vi "X_plus_h.vi"(5 "X":dbl[](array[numeric]), 7 "h":dbl, 9 "i":i32) -> (6 "Xi+h":dbl[](array[numeric]))   [LabVIEW 2017, in "NI_Gmath.lvlib"]
uses:
  <vilib>/gmath/NI_Gmath.lvlib
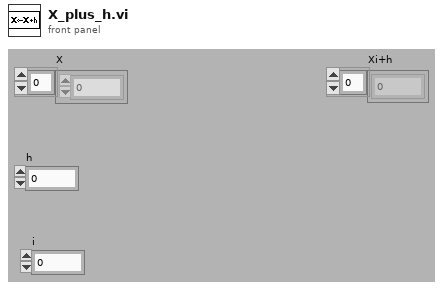
[diagram p1: front panel]
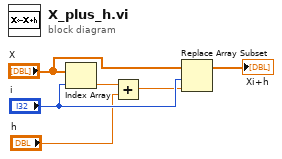
[diagram p0: block diagram]
diagram:
  n1 = Index Array(array="X", index="i") -> (element=w5:dbl)
  n2 = Add(x=w5, y="h") -> (x+y=w2:dbl)
  n3 = Replace Array Subset(array="X", new element=w2, index="i") -> (→"Xi+h":dbl[])
